vi "Integral x(t) PtByPt.vi"(2 "initialize":bool, 3 "dt":dbl=1.0 format="%0.2f", 4 "initial condition":dbl format="%0.2f", 5 "x":dbl format="%0.2f") -> (0 "error":i32, 1 "integral x(t)":dbl format="%0.2f")   [LabVIEW 2017, in "NI_PtbyPt.lvlib"]
doc: "Performs the discrete integration on <B>x</B>. You must sample <B>x</B> at regular intervals of <B>dt</B>."
uses:
  <vilib>/ptbypt/NI_PtbyPt.lvlib
  <vilib>/Analysis/NI_AALPro.lvlib
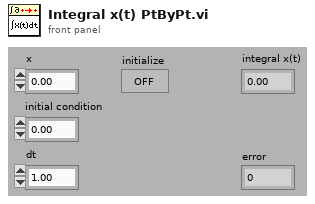
[diagram p1: front panel]
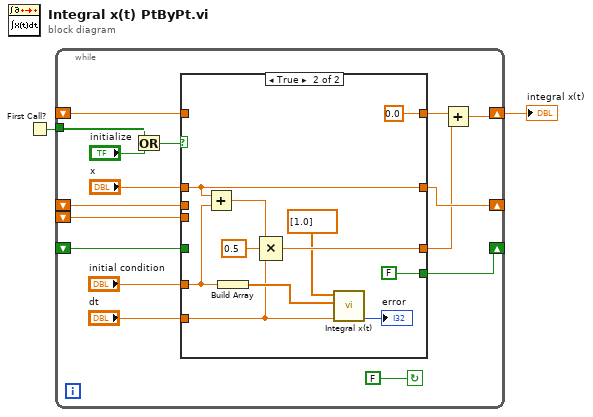
[diagram p0: block diagram]
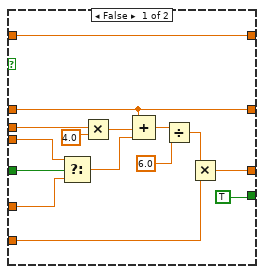
[diagram p2: hidden frame]
diagram:
  n1 = First Call?() -> (First Call?: T/F=w2:bool)
  n2 = while {
    shift-left: _ -> [w6]
    shift-right: [w3] -> w1
    tunnel: w2 -> [w15]
    shift-left: _ -> [w10]
    shift-right: [w18] -> _
    shift-left: _ -> [w8]
    shift-left: _ -> [w9]
    shift-right: [w12] -> _
    stop <- FALSE continue-if-true
    n3 = Or(x=w15, y="initialize") -> (x .or. y?=w14:bool)
    n4 = case shown="True" w14 {
      tunnel: [TRUE FALSE ("Boolean")] -> w18
      tunnel: "dt" -> [w32 w37]
      tunnel: "x" -> [w29 w41]
      tunnel: [w29 w41] -> w12
      tunnel: "initial condition" -> [w20 w34]
      tunnel: [w31 w44] -> w4
      tunnel: w10 -> [w22 _]
      tunnel: w9 -> [w33 _]
      tunnel: w8 -> [w21 _]
      tunnel: [w28 0.0] -> w5
      tunnel: w6 -> [w28 _]
      frame False {
        n5 = Select(t=w21, s=w22, f=w20) -> (s? t:f=w19:dbl)
        n6 = Multiply(x=w33, y=4.0) -> (x*y=w26:dbl)
        n7 = Compound Arithmetic op=ADD(w29, w26, w19) -> (w25:dbl)
        n8 = Divide(x=w25, y=6.0) -> (x/y=w23:dbl)
        n9 = Multiply(x=w23, y=w32) -> (x*y=w31:dbl)
      }
      frame True {
        n10 = Add(x=w41, y=w34) -> (x+y=w40:dbl)
        n11 = Build Array(w34) -> (w38:dbl[])
        n12 = Compound Arithmetic op=MULTIPLY(w40, 0.5 ("Input"), w37) -> (w44:dbl)
        n13 = call <vilib>:"Integral x(t).vi"("dt"=w37, "Initial Condition"=w38, "X"=dbl[] [1.0]) -> ("error"=→"error":i32)  [unwired: 7 in, 1 out]
      }
    }
    n14 = Add(x=w5, y=w4) -> (x+y=w3:dbl)
  }
  "integral x(t)" <- w1
